vi "myRIO v1.1 Register AI IRQ.vi"(3 "Hysteresis (0.02)":dbl=0.02, 4 "Callback VI Reference":T2, 5 "Allow Overwrite Operation? (F)":bool, 6 "Threshold":dbl=2.5, 7 "IRQ Number":u8, 8 "error in (no error)":errorcluster, 9 "Analog Interrupt Type":T3, 10 "Channel Name":string, 11 "Resource name":T1 caption="RIO Device") -> (0 "error out":errorcluster)   [LabVIEW 2021]
uses:
  <vilib>/myRIO/Common/Instrument Driver Framework/myRIO v1.0/IRQ/typedefs/AI IRQ Type.ctl
  <vilib>/myRIO/Common/Instrument Driver Framework/myRIO v1.0/IRQ/typedefs/Callback VI Ref.ctl
  <vilib>/userDefined/High Color/nirio_resource_hc.ctl
  <vilib>/myRIO/Common/Instrument Driver Framework/myRIO v1.0/IRQ/typedefs/IRQ Type.ctl
  <vilib>/myRIO/Common/Instrument Driver Framework/myRIO v1.0/IRQ/typedefs/IO IRQ Channels Enum.ctl
  <vilib>/myRIO/Common/Instrument Driver Framework/myRIO v1.0/IRQ/typedefs/myRIO v1.1 AI IRQ Channels Enum.ctl
  <vilib>/Utility/VariantDataType/GetNumericInfo.vi
  <vilib>/Utility/error.llb/Error Cluster From Error Code.vi
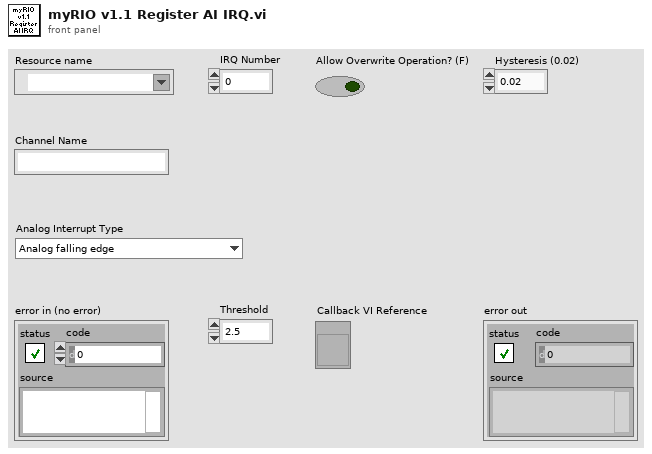
[diagram p1: front panel]
types:
  T1 = typedef "nirio_resource_hc.ctl" = tag
  T2 = typedef "Callback VI Ref.ctl" = refnum<vi>
  T3 = typedef "AI IRQ Type.ctl" = enum16{"Analog falling edge", "Analog rising edge"}
  T4 = typedef "IRQ Type.ctl" = enum16{"Timer", "Analog falling edge", "Analog rising edge", "Digital falling edge", "Digital rising edge", "Digital edge"}
  T5 = typedef "IO IRQ Channels Enum.ctl" = enum16{"Not Connected", "A/AI0 (Interrupt)", "A/AI1 (Interrupt)", "A/DIO0 (Interrupt)", "A/DIO1 (Interrupt)", "A/DIO2 (Interrupt)", "A/DIO3 (Interrupt)", "Button0 (Interrupt)", "B/AI0 (Interrupt)", "B/AI1 (Interrupt)", "B/DIO0 (Interrupt)", "B/DIO1 (Interrupt)", "B/DIO2 (Interrupt)", "B/DIO3 (Interrupt)"}
  T6 = typedef "myRIO v1.1 AI IRQ Channels Enum.ctl" = enum16{"Not Connected", "A/AI0 (Interrupt)", "A/AI1 (Interrupt)"}
  T7 = typedef "Generic FPGA Reference.ctl" = refnum<k20>
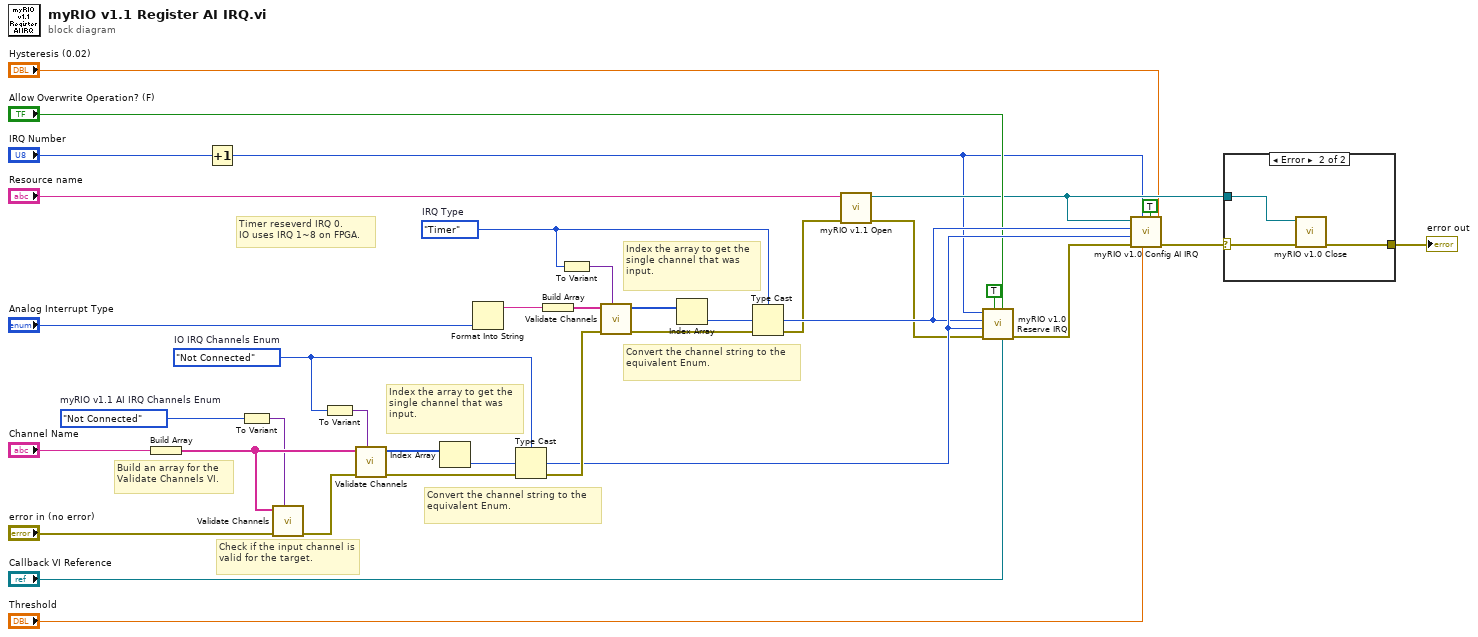
[diagram p0: block diagram]
diagram:
  w23 = IRQ_Type."Timer"  # IRQ Type
  w27 = IO_IRQ_Channels_Enum."Not Connected"  # IO IRQ Channels Enum
  w30 = myRIO_v1.1_AI_IRQ_Channels_Enum."Not Connected"  # myRIO v1.1 AI IRQ Channels Enum
  # "Timer reseverd IRQ 0.\nIO uses IRQ 1~8 on FPGA."
  # "Index the array to get the single channel that was input."
  # "Convert the channel string to the equivalent Enum."
  # "Index the array to get the single channel that was input."
  # "Build an array for the Validate Channels VI."
  # "Convert the channel string to the equivalent Enum."
  # "Check if the input channel is valid for the target."
  n1 = Build Array("Channel Name") -> (w33:string[])
  n2 = Increment(x="IRQ Number") -> (x+1=w2:u8)
  n3 = To Variant(anything=w30) -> (Variant=w29:variant)
  n4 = call <vilib>:"Validate Channels.vi"("Channels Enum Variant"=w29, "error in (no error)"="error in (no error)", "Channel Names"=w33) -> ("error out"=w4:errorcluster)  [unwired: 7 in, 1 out]
  n5 = To Variant(anything=w27) -> (Variant=w28:variant)
  n6 = call <vilib>:"Validate Channels.vi"("Channels Enum Variant"=w28, "error in (no error)"=w4, "Channel Names"=w33) -> ("error out"=w21:errorcluster, "Index Array"=w34:u16[])  [unwired: 7 in]
  n7 = Index Array(array=w34) -> (element=w35:u16)  [unwired: 1 in]
  n8 = Format Into String("Analog Interrupt Type") -> (resulting string=w5:string)  [unwired: 3 in, 1 out]
  n9 = Type Cast(type=w27, x=w35) -> (*(type *) &x=w18:T5)
  n10 = Build Array(w5) -> (w22:string[])
  n11 = To Variant(anything=w23) -> (Variant=w26:variant)
  n12 = call <vilib>:"Validate Channels.vi"("Channels Enum Variant"=w26, "error in (no error)"=w21, "Channel Names"=w22) -> ("error out"=w9:errorcluster, "Index Array"=w25:u16[])  [unwired: 7 in]
  n13 = Index Array(array=w25) -> (element=w24:u16)  [unwired: 1 in]
  n14 = Type Cast(type=w23, x=w24) -> (*(type *) &x=w17:T4)
  n15 = call <vilib>:"myRIO v1.1 Open.vi"("error in (no error)"=w9, "Resource name"="Resource name") -> ("error out"=w8:errorcluster, "myRIO FPGA Ref Out"=w10:T7)  [unwired: 8 in]
  n16 = call <vilib>:"myRIO v1.0 Reserve IRQ.vi"("Callback VI Ref"="Callback VI Reference", "Allow Overwrite? (F)"="Allow Overwrite Operation? (F)", "Is Reserve?"=TRUE, "error in (no error)"=w8, "IO IRQ Channels Enum"=w18, "IRQ Type"=w17, "IRQ Number"=w2) -> ("error out"=w19:errorcluster)  [unwired: 3 in, 1 out]
  n17 = call <vilib>:"myRIO v1.0 Config AI IRQ.vi"("Hysteresis"="Hysteresis (0.02)", "Enable IRQ?"=TRUE, "Threshold"="Threshold", "IRQ Number"=w2, "error in (no error)"=w19, "IO IRQ Channels Enum"=w18, "IRQ Type"=w17, "myRIO FPGA Ref In"=w10) -> ("error out"=w13:errorcluster)  [unwired: 3 in]
  n18 = case shown="Error" w13 {
    selector: w13 -> [w36 w39]
    tunnel: w10 -> [_ w37]
    tunnel: [w36 w38] -> w12
    frame No Error {
    }
    frame Error {
      n19 = call <vilib>:"myRIO v1.0 Close.vi"("error in (no error)"=w39, "myRIO FPGA Ref In"=w37) -> ("error out"=w38:errorcluster)  [unwired: 9 in]
    }
  }
  "error out" <- w12
